vi "Rolling buffer.vi"(9 "Value in":dbl, 10 "Reset buffer":bool, 11 "Buffer length (points)":i32) -> (1 "Rolling buffer":dbl[](array[numeric]))   [LabVIEW 2013]
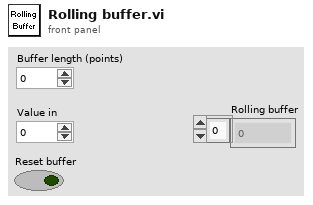
[diagram p1: front panel]
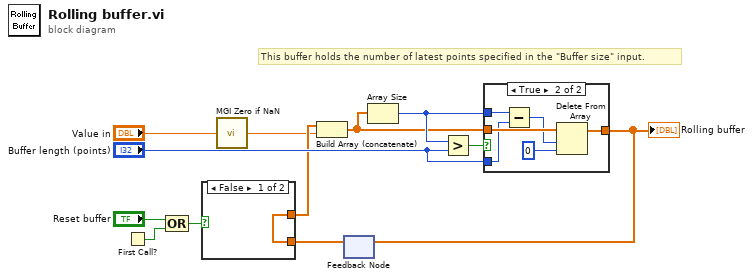
[diagram p0: block diagram]
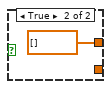
[diagram p2: hidden frame]
diagram:
  # "This buffer holds the number of latest points specified in the \"Buffer size\" input."
  n1 = First Call?() -> (First Call?: T/F=w3:bool)
  n2 = Compound Arithmetic op=OR("Reset buffer", w3) -> (w4:bool)
  n3 = call "MGI Zero if NaN.vi"("Number In"="Value in") -> ("Number Out"=w1:dbl)
  n4 = feedback #1() -> (w6:dbl[])  [unwired: 1 in]
  n5 = case shown="False" w4 {
    tunnel: [w13 dbl[] []] -> w7
    tunnel: w6 -> [w13 _]
    frame False {
    }
    frame True {
    }
  }
  n6 = Build Array (concatenate)(w7, w1) -> (w9:dbl[])
  n7 = Array Size(array=w9) -> (size(s)=w10:i32)
  n8 = Greater?(x=w10, y="Buffer length (points)") -> (0:w8:bool)
  n9 = case shown="True" w8 {
    tunnel: w9 -> [w15 w21]
    tunnel: [w15 w20] -> w12
    tunnel: w10 -> [_ w18]
    tunnel: "Buffer length (points)" -> [_ w17]
    frame False {
    }
    frame True {
      n10 = Subtract(x=w18, y=w17) -> (x-y=w16:i32)
      n11 = Delete From Array(array=w21, length=w16, index=0) -> (array with subset deleted=w20:dbl[])  [unwired: 1 out]
    }
  }
  "Rolling buffer" <- w12
  n12 = feedback-in #1(w12) -> ()
